vi "getFont.vi"(8 "error in (no error)":errorcluster, 11 "Theme in":refnum<class "Theme.lvclass">) -> (0 "error out":errorcluster, 2 "Colors":T1, 3 "Theme out":refnum<class "Theme.lvclass">)   [LabVIEW 2017, in "Theme.lvlib" / "Theme.lvclass"]
uses:
  Theme.lvclass
  Theme.Font/Font.ctl
  Theme.lvclass/Theme.ctl
  Theme.Font/Theme.Font.lvclass/Theme.Font.ctl
  Theme.Font/getSize.vi
  Theme.Font/getShrinkSize.vi
  Theme.Font/getName.vi
  Theme.Font/getPasswordDisplay.vi
  Theme.Colors/Theme.Colors.lvclass
  Theme.Font/Theme.Font.lvclass
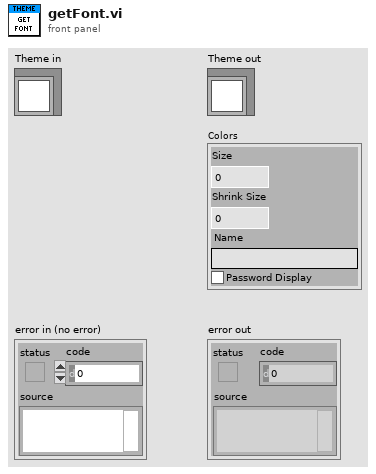
[diagram p1: front panel]
types:
  T1 = typedef "Theme.lvlib/Theme.Font.lvclass/Font.ctl" = cluster{"Size":u32, "Shrink Size":u32, "Name":string, "Password Display":bool}
  T2 = typedef "Theme.lvlib/Theme.lvclass/Private Data.ctl" = cluster{"Colors":refnum<class "Theme.Colors.lvclass">, "Font":refnum<class "Theme.Font.lvclass">}
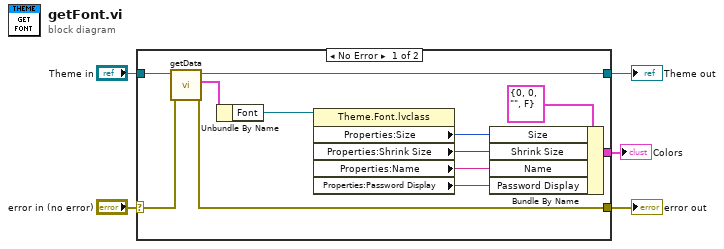
[diagram p0: block diagram]
diagram:
  n1 = case shown="No Error" "error in (no error)" {
    selector: "error in (no error)" -> [w13 w19]
    tunnel: [w12 w19] -> w4
    tunnel: [w16 w18] -> w2
    tunnel: "Theme in" -> [w17 w18]
    tunnel: [w7 _] -> w1
    frame No Error {
      n2 = call "getData.vi"("error in (no error)"=w13, "Theme in"=w17) -> ("error out"=w12:errorcluster, "Theme"=w15:T2, "Theme out"=w16:refnum<class "Theme.lvclass">)  [unwired: 7 in]
      n3 = Unbundle By Name(w15) -> ("Font"=w14:refnum<class "Theme.Font.lvclass">)
      n4 = property class="Theme.Font.lvclass"(reference=w14) -> ("Properties:Size"=w8:u32, "Properties:Shrink Size"=w9:u32, "Properties:Name"=w10:string, "Properties:Password Display"=w6:bool)  [unwired: 1 in, 2 out]
      n5 = Bundle By Name(cluster=T1 {"Size"=0, "Shrink Size"=0, "Name"="", "Password Display"=FALSE} ("Filled Text Fields.Theme.Font"), "Size"=w8, "Shrink Size"=w9, "Name"=w10, "Password Display"=w6) -> (w7:T1)
    }
    frame Error {
    }
  }
  "error out" <- w4
  "Theme out" <- w2
  "Colors" <- w1
